vi "Query Active DUT IMS.vi"(8 "error in (no error)":errorcluster, 10 "SIM Slot (1)":i32=1, 11 "VISA resource name":refnum<visa-resource-name>) -> (0 "error out":errorcluster, 2 "IMS":bool, 3 "VISA resource name out":refnum<visa-resource-name>)   [LabVIEW 2015, in "Rohde&Schwarz CMXP Base.lvlib"]
doc: "Queries the reported IMS capabilities of the active DUT.\n\nAttribute:\nRSCMXPBASE_ATTR_ACTIVE_DUT_IMS\n\nRemote-control command:\nSENSe:DUT:MODem<ModemIdx>:CAPability:REPorted:IMS?"
uses:
  <instrlib>/Rohde&Schwarz CMXP Base/Rohde&Schwarz CMXP Base.lvlib
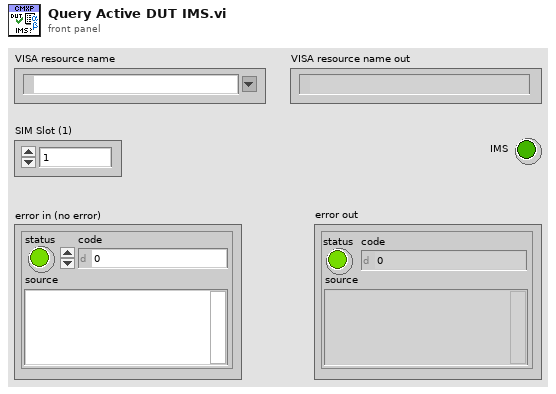
[diagram p1: front panel]
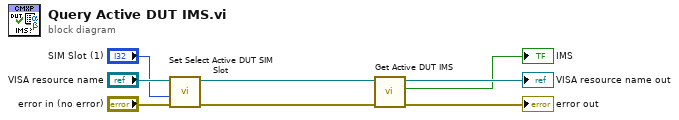
[diagram p0: block diagram]
diagram:
  n1 = call "Set Select Active DUT SIM Slot"("error in (no error)"="error in (no error)", "Select Active DUT SIM Slot (0)"="SIM Slot (1)", "instrument handle"="VISA resource name") -> ("error out"=w4:errorcluster, "instrument handle out"=w3:refnum<visa-resource-name>)  [unwired: 7 in]
  n2 = call "Get Active DUT IMS"("error in (no error)"=w4, "instrument handle"=w3) -> ("error out"=→"error out":errorcluster, "Active DUT IMS"=→"IMS":bool, "instrument handle out"=→"VISA resource name out":refnum<visa-resource-name>)  [unwired: 7 in]
